vi "Data To SingleElementsArray_jkism.vi"(6 "Seperator(/)":string="/", 8 "error in (no error)":errorcluster, 10 "parentUrl":string, 11 "Cluster":variant) -> (0 "error out":errorcluster, 2 "Full NameList":string[](array[string]), 3 "DataElementArray":variant[](array[variant]))   [LabVIEW 2017, in "JKISM++ API String Arguments Support.lvlib"]
doc: "This VI converts a Cluster to a DataElementArray with each elements specified by parentUrl and Seperator in the form of Tree Description."
uses:
  JKISM++ API String Arguments Support.lvlib
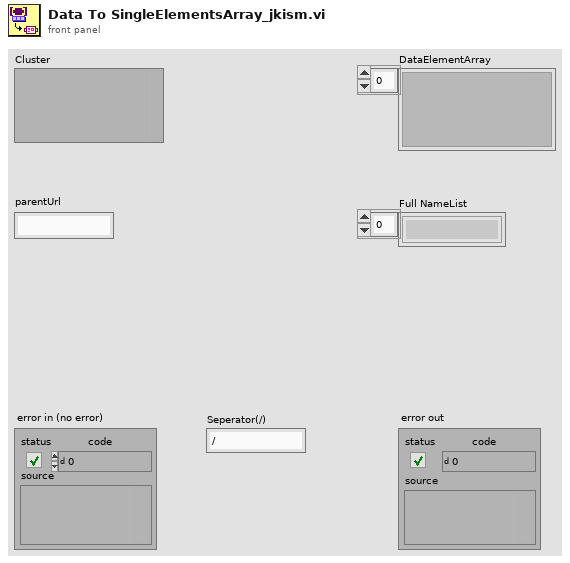
[diagram p1: front panel]
types:
  T1 = typedef "Type Descriptor Enumeration__ogtk.ctl" = enum8{"<Null>", "I8", "I16", "I32", "I64", "U8", "U16", "U32", "U64", "SGL", "DBL", "EXT", "CSG", "CDB", "CXT", "0x0F", "0x10", "0x11", "0x12", "0x13", "0x14", "Enum U8", "Enum U16", "Enum U32", "Enum U64", "SGL PQ", "DBL PQ", "EXT PQ", "CSG PQ", "CDB PQ", "CXT PQ", "0x1F", "0x20", "Boolean", "0x22", "0x23", "0x24", "0x25", "0x26", "0x27", "0x28", "0x29", "0x2A", "0x2B", "0x2C", "0x2D", "0x2E", "0x2F", "String", "0x31", "Path", "Pict", "0x34", "0x35", "0x36", "DAQ", "0x38", "0x39", "0x3A", "0x3B", "0x3C", "0x3D", "0x3E", "0x3F", "Array", "0x41", "0x42", "0x43", "0x44", "0x45", "0x46", "0x47", "0x48", "0x49", "0x4A", "0x4B", "0x4C", "0x4D", "0x4E", "0x4F", "Cluster", "0x51", "0x52", "Variant", "Waveform", "0x55", "0x56", "0x57", "0x58", "0x59", "0x5A", "0x5B", "0x5C", "0x5D", "0x5E", "Fixed Point", "0x60", "0x61", "0x62", "0x63", "0x64", "0x65", "0x66", "0x67", "0x68", "0x69", "0x6A", "0x6B", "0x6C", "0x6D", "0x6E", "0x6F", "Refnum", "0x71", "0x72", "Set Collection", "Map Collection"}
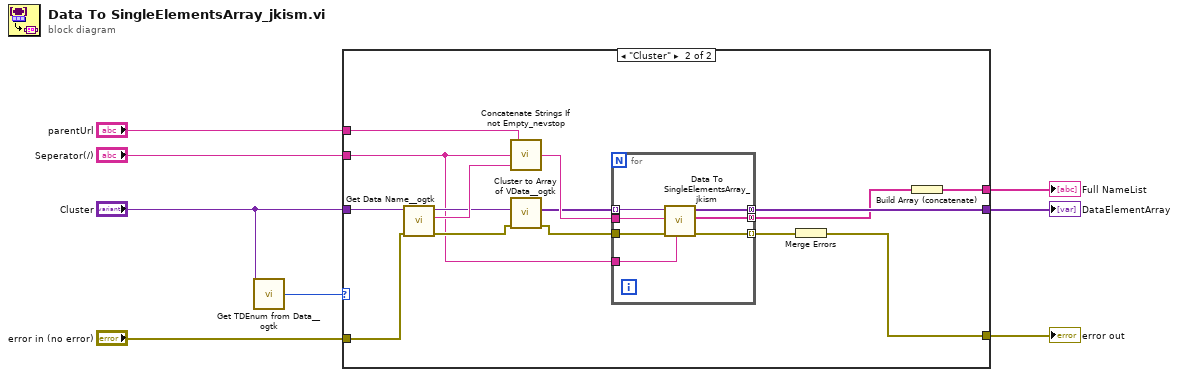
[diagram p0: block diagram]
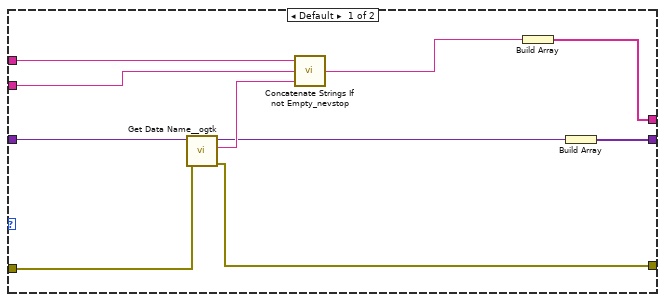
[diagram p2: hidden frame]
diagram:
  n1 = call "Get TDEnum from Data__ogtk.vi"("Data"="Cluster") -> ("Type Descriptor Enumeration"=w8:T1)  [unwired: 4 in]
  n2 = case shown="\"Cluster\"" w8 {
    tunnel: "Cluster" -> [w18 w33]
    tunnel: "parentUrl" -> [w17 w30]
    tunnel: "error in (no error)" -> [w15 w21]
    tunnel: [w11 w31] -> w4
    tunnel: [w14 w26] -> w3
    tunnel: [w12 w24] -> w2
    tunnel: "Seperator(/)" -> [w9 w19]
    frame Default {
      n3 = call "Get Data Name__ogtk.vi"("error in (no error)"=w15, "Data"=w18) -> ("error out"=w11:errorcluster, "Data Name"=w16:string, "Data dup"=w10:variant)  [unwired: 7 in]
      n4 = call "Concatenate Strings If not Empty_nevstop.vi"("String"=w16, "seperator(:)"=w9, "prefix"=w17) -> ("result"=w13:string)  [unwired: 2 in]
      n5 = Build Array(w13) -> (w12:string[])
      n6 = Build Array(w10) -> (w14:variant[])
    }
    frame "Cluster" {
      n7 = call "Get Data Name__ogtk.vi"("error in (no error)"=w21, "Data"=w33) -> ("error out"=w22:errorcluster, "Data Name"=w29:string, "Data dup"=w23:variant)  [unwired: 7 in]
      n8 = call "Concatenate Strings If not Empty_nevstop.vi"("String"=w29, "seperator(:)"=w19, "prefix"=w30) -> ("result"=w28:string)  [unwired: 2 in]
      n9 = call "Cluster to Array of VData__ogtk.vi"("error in (no error)"=w22, "Cluster"=w23) -> ("error out"=w20:errorcluster, "Array of VData"=w27:variant[])  [unwired: 8 in]
      n10 = for {
        tunnel: w27 -> [w40] mode=indexing
        tunnel: w28 -> [w39]
        tunnel: [w38] -> w26 mode=concatenating
        tunnel: w20 -> [w37]
        tunnel: [w36] -> w32 mode=indexing
        tunnel: [w35] -> w25 mode=concatenating
        tunnel: w19 -> [w34]
        n11 = call "Data To SingleElementsArray_jkism.vi"("Seperator(/)"=w34, "error in (no error)"=w37, "parentUrl"=w39, "Cluster"=w40) -> ("error out"=w36:errorcluster, "Full NameList"=w35:string[], "DataElementArray"=w38:variant[])  [unwired: 5 in]
      }
      n12 = Merge Errors(w32) -> (w31:errorcluster)
      n13 = Build Array (concatenate)(w25) -> (w24:string[])
    }
  }
  "Full NameList" <- w2
  "error out" <- w4
  "DataElementArray" <- w3
